vi "Measure.vi"(8 "error in":errorcluster, 10 "Controle":T1, 11 "map reference in":refnum<data-value>) -> (0 "error out":errorcluster, 2 "Indicator":T1, 3 "map reference out":refnum<data-value>, 4 "Intensity Graph":dbl[][](graph), 6 "XY Graph":cluster{dbl[], dbl[]}[](graph))   [LabVIEW 2012]
uses:
  <vilib>/robotics/Navigation/shared/WorldMap/OccupancyGridWorldMap/NI_Robotics_OccupancyGridWorldMap.lvclass
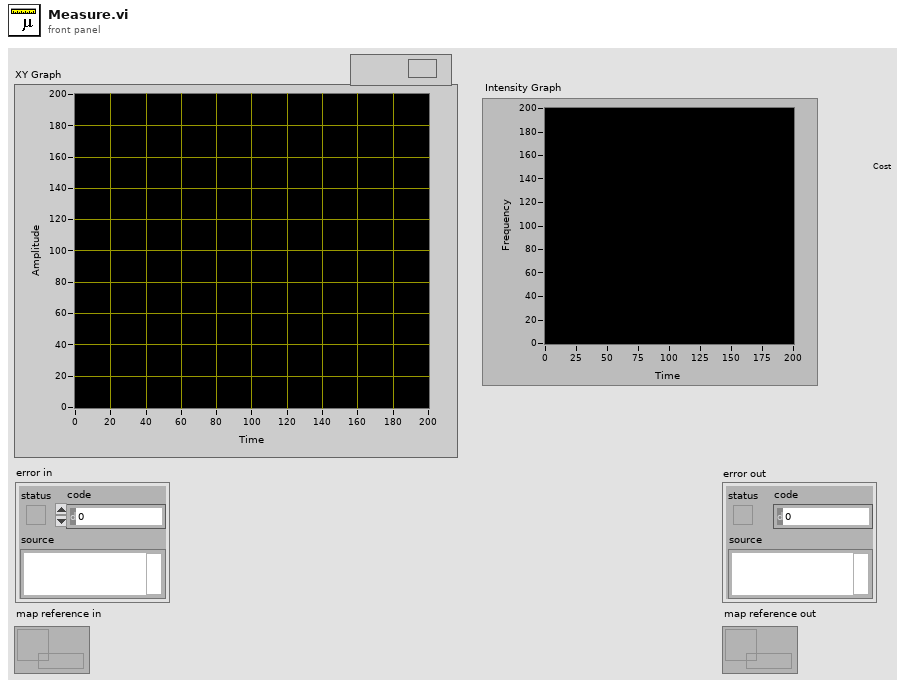
[diagram p1: front panel]
types:
  T1 = cluster{"Resolution":i32, "Scale":dbl, "Data":cluster{"GPS Data":cluster{"Latitude":dbl, "Longitude":dbl, "Altitude":dbl, "Velocity, Correction & SET":cluster{"Velocity North":dbl, "Velocity East":dbl, "Velocity Up":dbl, "Ellipsoidal Height":dbl, "GDOP":sgl, "PDOP":sgl, "HDOP":sgl, "VDOP":sgl, "TDOP":sgl, "Horizontal Figure of Merit":u8, "Time Figure of Merit":u8, "Max dGPS Age":sgl, "Extended Navigation Mode":u8, "Antenna Height Adjustment ":dbl, "SET North":i32, "SET East":i32, "SET Up":i32}, "Time":cluster{"GPS Week":u16, "GPS Time of Week":sgl}, "Satellites Used":i32[]}, "IMU Data":cluster{"Position":cluster{"Roll":dbl, "Pitch":dbl, "Yaw":dbl}, "Orientation Matrix":dbl[][], "Magnetic Field":cluster{"Z-Axis Magnetic Field":dbl, "Y-Axis Magnetic Field":dbl, "X-Axis Magnetic Field":dbl}, "Acceleration":cluster{"Z-Axis Acceleration":dbl, "Y-Axis Acceleration":dbl, "X-Axis Acceleration":dbl}, "Angular Rate":cluster{"X-Axis Angular Rate":dbl, "Y-Axis Angular Rate":dbl, "Z-Axis Angular Rate":dbl}, "Quaternion":dbl[]}, "LIDAR Data":cluster{"Magnitude":dbl[], "Direction":dbl[]}, "Telemetry":cluster{"Voltage":cluster{sgl, sgl, sgl}, "Encoder Speed":cluster{i32, i32}, "Temps":cluster{"IC Temp (C)":i32, "Ch1 Temp (C)":i32, "Ch2 Temp (C)":i32}, "Current":cluster{dbl, dbl, dbl, dbl}}, "Lines":cluster{"Start Point":cluster{"X":sgl, "Y":sgl}, "End Point":cluster{"X":sgl, "Y":sgl}, "Length":dbl, "Orientation":dbl, "Score":dbl}[]}, "initialized array":dbl[][]}
  T2 = cluster{"Voltage":cluster{sgl, sgl, sgl}, "Encoder Speed":cluster{i32, i32}, "Temps":cluster{"IC Temp (C)":i32, "Ch1 Temp (C)":i32, "Ch2 Temp (C)":i32}, "Current":cluster{dbl, dbl, dbl, dbl}}
  T3 = cluster{"Latitude":dbl, "Longitude":dbl, "Altitude":dbl, "Velocity, Correction & SET":cluster{"Velocity North":dbl, "Velocity East":dbl, "Velocity Up":dbl, "Ellipsoidal Height":dbl, "GDOP":sgl, "PDOP":sgl, "HDOP":sgl, "VDOP":sgl, "TDOP":sgl, "Horizontal Figure of Merit":u8, "Time Figure of Merit":u8, "Max dGPS Age":sgl, "Extended Navigation Mode":u8, "Antenna Height Adjustment ":dbl, "SET North":i32, "SET East":i32, "SET Up":i32}, "Time":cluster{"GPS Week":u16, "GPS Time of Week":sgl}, "Satellites Used":i32[]}
  T4 = cluster{"Position":cluster{"Roll":dbl, "Pitch":dbl, "Yaw":dbl}, "Orientation Matrix":dbl[][], "Magnetic Field":cluster{"Z-Axis Magnetic Field":dbl, "Y-Axis Magnetic Field":dbl, "X-Axis Magnetic Field":dbl}, "Acceleration":cluster{"Z-Axis Acceleration":dbl, "Y-Axis Acceleration":dbl, "X-Axis Acceleration":dbl}, "Angular Rate":cluster{"X-Axis Angular Rate":dbl, "Y-Axis Angular Rate":dbl, "Z-Axis Angular Rate":dbl}, "Quaternion":dbl[]}
  T5 = cluster{"Start Point":cluster{"X":sgl, "Y":sgl}, "End Point":cluster{"X":sgl, "Y":sgl}, "Length":dbl, "Orientation":dbl, "Score":dbl}[]
  T6 = cluster{"GPS Data":cluster{"Latitude":dbl, "Longitude":dbl, "Altitude":dbl, "Velocity, Correction & SET":cluster{"Velocity North":dbl, "Velocity East":dbl, "Velocity Up":dbl, "Ellipsoidal Height":dbl, "GDOP":sgl, "PDOP":sgl, "HDOP":sgl, "VDOP":sgl, "TDOP":sgl, "Horizontal Figure of Merit":u8, "Time Figure of Merit":u8, "Max dGPS Age":sgl, "Extended Navigation Mode":u8, "Antenna Height Adjustment ":dbl, "SET North":i32, "SET East":i32, "SET Up":i32}, "Time":cluster{"GPS Week":u16, "GPS Time of Week":sgl}, "Satellites Used":i32[]}, "IMU Data":cluster{"Position":cluster{"Roll":dbl, "Pitch":dbl, "Yaw":dbl}, "Orientation Matrix":dbl[][], "Magnetic Field":cluster{"Z-Axis Magnetic Field":dbl, "Y-Axis Magnetic Field":dbl, "X-Axis Magnetic Field":dbl}, "Acceleration":cluster{"Z-Axis Acceleration":dbl, "Y-Axis Acceleration":dbl, "X-Axis Acceleration":dbl}, "Angular Rate":cluster{"X-Axis Angular Rate":dbl, "Y-Axis Angular Rate":dbl, "Z-Axis Angular Rate":dbl}, "Quaternion":dbl[]}, "LIDAR Data":cluster{"Magnitude":dbl[], "Direction":dbl[]}, "Telemetry":cluster{"Voltage":cluster{sgl, sgl, sgl}, "Encoder Speed":cluster{i32, i32}, "Temps":cluster{"IC Temp (C)":i32, "Ch1 Temp (C)":i32, "Ch2 Temp (C)":i32}, "Current":cluster{dbl, dbl, dbl, dbl}}, "Lines":cluster{"Start Point":cluster{"X":sgl, "Y":sgl}, "End Point":cluster{"X":sgl, "Y":sgl}, "Length":dbl, "Orientation":dbl, "Score":dbl}[]}
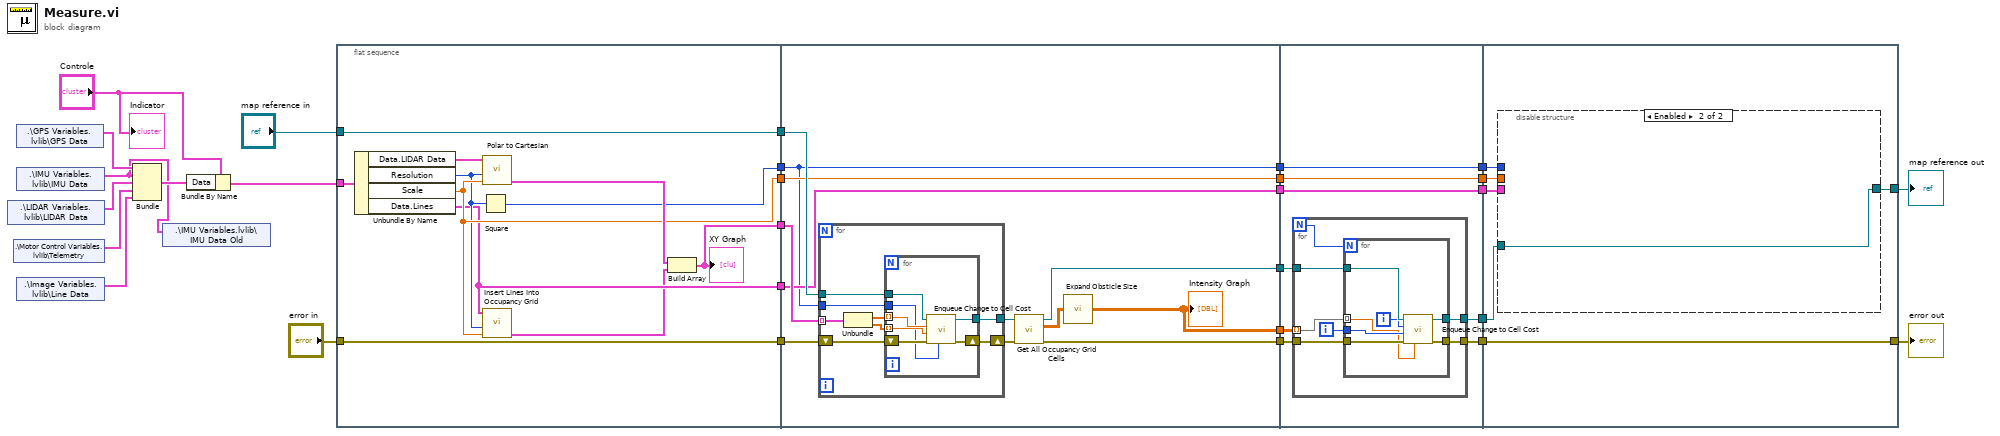
[diagram p0: block diagram]
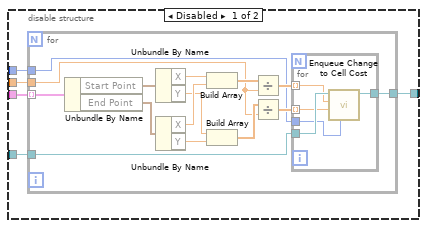
[diagram p2: hidden frame]
diagram:
  n1 = shared-variable ".\\LIDAR Variables.lvlib\\LIDAR Data"() -> (w24:cluster{"Magnitude":dbl[], "Direction":dbl[]})  [unwired: 1 in, 1 out]
  n2 = shared-variable ".\\Motor Control Variables.lvlib\\Telemetry"() -> (w23:T2)  [unwired: 1 in, 1 out]
  n3 = shared-variable ".\\GPS Variables.lvlib\\GPS Data"() -> (w25:T3)  [unwired: 1 in, 1 out]
  n4 = shared-variable ".\\IMU Variables.lvlib\\IMU Data"() -> (w1:T4)  [unwired: 1 in, 1 out]
  n5 = shared-variable ".\\Image Variables.lvlib\\Line Data"() -> (w13:T5)  [unwired: 1 in, 1 out]
  n6 = Bundle("GPS Data"=w25, "IMU Data"=w1, "LIDAR Data"=w24, "Telemetry"=w23, "Lines"=w13) -> (w22:T6)  [unwired: 1 in]
  n7 = shared-variable ".\\IMU Variables.lvlib\\IMU Data Old"(w1) -> ()  [unwired: 1 in, 1 out]
  n8 = Bundle By Name(cluster="Controle", "Data"=w22) -> (w21:T1)
  n9 = flat-sequence {
    tunnel: "map reference in" -> [w40]
    tunnel: [w40] -> w26
    tunnel: w21 -> [w39]
    tunnel: [w36] -> w19
    tunnel: [w31] -> w18
    tunnel: [w35] -> w17
    tunnel: [w33] -> w16
    tunnel: "error in" -> [w32]
    tunnel: [w32] -> w14
    tunnel: w26 -> [w48]
    tunnel: w19 -> [w51]
    tunnel: [w50] -> w12
    tunnel: [w49] -> w10
    tunnel: [w45] -> w8
    tunnel: w18 -> [w45]
    tunnel: [w44] -> w6
    tunnel: w17 -> [w44]
    tunnel: w16 -> [w43]
    tunnel: [w43] -> w4
    tunnel: w14 -> [w42]
    tunnel: [w41] -> w2
    tunnel: w12 -> [w72]
    tunnel: [w71] -> w11
    tunnel: w10 -> [w70]
    tunnel: [w69] -> w9
    tunnel: w8 -> [w75]
    tunnel: [w75] -> w7
    tunnel: w6 -> [w74]
    tunnel: [w74] -> w5
    tunnel: w4 -> [w73]
    tunnel: [w73] -> w3
    tunnel: w2 -> [w68]
    tunnel: [w95] -> w28
    tunnel: [w91] -> w29
    tunnel: w11 -> [w92]
    tunnel: w9 -> [w95]
    tunnel: w7 -> [w94]
    tunnel: w5 -> [w93]
    tunnel: w3 -> [w90]
    frame #0 {
      n10 = Unbundle By Name(w39) -> ("Data.LIDAR Data"=w38:cluster{"Magnitude":dbl[], "Direction":dbl[]}, "Resolution"=w34:i32, "Scale"=w35:dbl, "Data.Lines"=w31:T5)
      n11 = Square(x=w34) -> (x^2=w33:i32)
      n12 = call "Polar to Cartesian.vi"("Scale"=w35, "Resulotion"=w34, "LIDAR Data"=w38) -> ("XY"=w37:cluster{dbl[], dbl[]})  [unwired: 7 in, 1 out]
      n13 = call "Insert Lines Into Occupancy Grid.vi"("Scale"=w35, "Resolution"=w34, "Lines In"=w31) -> ("XY"=w30:cluster{dbl[], dbl[]})  [unwired: 7 in, 1 out]
      n14 = Build Array(w37, w30) -> (w36:cluster{dbl[], dbl[]}[])
      "XY Graph" <- w36
    }
    frame #1 {
      n15 = for {
        tunnel: [w60] -> w52
        tunnel: w51 -> [w57] mode=indexing
        tunnel: w48 -> [w56]
        shift-right: [w54] -> w47
        shift-left: w42 -> [w55]
        tunnel: w43 -> [w53]
        n16 = Unbundle(w57) -> (w58:dbl[], w59:dbl[])
        n17 = for {
          tunnel: w58 -> [w66] mode=indexing
          tunnel: w59 -> [w67] mode=indexing
          tunnel: w56 -> [w65]
          tunnel: [w64] -> w60
          shift-right: [w62] -> w54
          shift-left: w55 -> [w63]
          tunnel: w53 -> [w61]
          n18 = call <vilib>:"Enqueue Change to Cell Cost.vi"("cost"=w61, "error in (no error)"=w63, "y"=w67, "x"=w66, "map reference in"=w65) -> ("error out"=w62:errorcluster, "map reference out"=w64:refnum<data-value>)  [unwired: 5 in]
        }
      }
      n19 = call <vilib>:"Get All Occupancy Grid Cells.vi"("error in (no error)"=w47, "map reference in"=w52) -> ("error out"=w49:errorcluster, "occupancy grid"=w46:dbl[][], "map reference out"=w50:refnum<data-value>)  [unwired: 7 in]
      n20 = call "Expand Obsticle Size.vi"("Map In"=w46) -> ("Map Out"=w41:dbl[][])
      "Intensity Graph" <- w41
    }
    frame #2 {
      n21 = for {
        N -> [w77]
        tunnel: w72 -> [w82]
        tunnel: [w81] -> w71
        tunnel: w70 -> [w79]
        tunnel: [w78] -> w69
        tunnel: w68 -> [w76] mode=indexing
        i -> [w80]
        n22 = for {
          N: w77 -> [_]
          tunnel: w82 -> [w89]
          tunnel: [w88] -> w81
          tunnel: w80 -> [w86]
          tunnel: w79 -> [w85]
          tunnel: [w84] -> w78
          tunnel: w76 -> [w83] mode=indexing
          i -> [w87]
          n23 = call <vilib>:"Enqueue Change to Cell Cost.vi"("cost"=w83, "error in (no error)"=w85, "y"=w86, "x"=w87, "map reference in"=w89) -> ("error out"=w84:errorcluster, "map reference out"=w88:refnum<data-value>)  [unwired: 5 in]
        }
      }
    }
    frame #3 {
      n24 = disable-structure shown="Enabled" {
        disable-tunnel: w94 -> [w100 _]
        disable-tunnel: w93 -> [w99 _]
        disable-tunnel: w92 -> [w98 w121]
        disable-tunnel: [w97 w121] -> w91
        disable-tunnel: w90 -> [w96 _]
        frame Disabled {
          n25 = for {
            tunnel: w100 -> [w115] mode=indexing
            tunnel: w99 -> [w106]
            tunnel: w98 -> [w103]
            tunnel: [w102] -> w97
            tunnel: w96 -> [w101]
            n26 = Unbundle By Name(w115) -> ("Start Point"=w113:cluster{"X":sgl, "Y":sgl}, "End Point"=w114:cluster{"X":sgl, "Y":sgl})
            n27 = Unbundle By Name(w113) -> ("X"=w112:sgl, "Y"=w110:sgl)
            n28 = Unbundle By Name(w114) -> ("X"=w111:sgl, "Y"=w109:sgl)
            n29 = Build Array(w112, w111) -> (w108:sgl[])
            n30 = Build Array(w110, w109) -> (w107:sgl[])
            n31 = Divide(x=w108, y=w106) -> (x/y=w105:dbl[])
            n32 = Divide(x=w107, y=w106) -> (x/y=w104:dbl[])
            n33 = for {
              tunnel: w105 -> [w118] mode=indexing
              tunnel: w104 -> [w117] mode=indexing
              tunnel: w103 -> [w119]
              tunnel: [w120] -> w102
              tunnel: w101 -> [w116]
              n34 = call <vilib>:"Enqueue Change to Cell Cost.vi"("cost"=w116, "y"=w117, "x"=w118, "map reference in"=w119) -> ("map reference out"=w120:refnum<data-value>)  [unwired: 6 in, 1 out]
            }
          }
        }
        frame Enabled {
        }
      }
    }
  }
  "map reference out" <- w29
  "error out" <- w28
  "Indicator" <- "Controle"
